vi "To Generic.vi"(8 "error in (no error)":errorcluster, 11 "NI DMM Calibration Data in":refnum<class "NI DMM Calibration Data.lvclass">) -> (0 "error out":errorcluster, 2 "Generic Data":refnum<class "Generic Data.lvclass">[](array[class]), 3 "Data Name":string[](array[string]))   [LabVIEW 2020, in "NI DMM Driver.lvlib" / "NI DMM Calibration Data.lvclass"]
doc: "Present private data as an array of named generic data elements."
uses:
  NI DMM Calibration Data.lvclass
  PPL/HDH.Data.Generic.lvlibp/Generic Data/Generic Data.lvclass
  NI DMM Calibration Data.lvclass/NI DMM Calibration Data.ctl
  PPL/HDH.Data.Generic.lvlibp/Generic Data/Time Stamp/Time Stamp.lvclass
  C:/Current projects/WS/PPL/HDH.Data.Generic.lvlibp/Generic Data/Generic Data.lvclass
  PPL/HDH.Data.Generic.lvlibp/Generic Data/String/String.lvclass
  PPL/HDH.Data.Generic.lvlibp/Generic Data/Boolean/Boolean.lvclass
  PPL/HDH.Data.Generic.lvlibp/Generic Data/Double/Double.lvclass
  PPL/HDH.Data.Generic.lvlibp/Data.lvclass
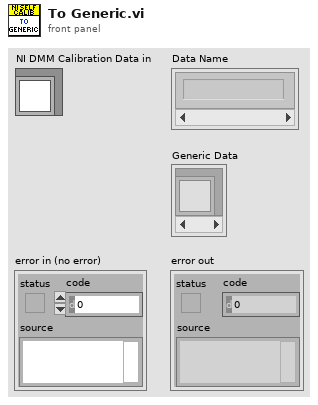
[diagram p1: front panel]
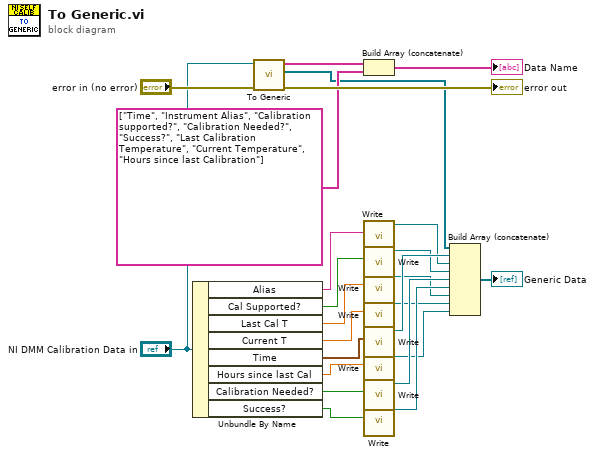
[diagram p0: block diagram]
diagram:
  n1 = Unbundle By Name("NI DMM Calibration Data in") -> ("Alias"=w13:string, "Cal Supported?"=w14:bool, "Last Cal T"=w6:dbl, "Current T"=w4:dbl, "Time"=w16:timestamp, "Hours since last Cal"=w2:dbl, "Calibration Needed?"=w10:bool, "Success?"=w9:bool)
  n2 = call-parent "To Generic.vi"("error in (no error)"="error in (no error)", "Data in"="NI DMM Calibration Data in") -> ("error out"=→"error out":errorcluster, "Generic Data"=w19:refnum<class "Generic Data.lvclass">[], "Data Name"=w23:string[])  [unwired: 7 in]
  n3 = Build Array (concatenate)(w23, string[] ["Time", "Instrument Alias", "Calibration supported?", "Calibration Needed?", "Success?", "Last Calibration Temperature", "Current Temperature", "Hours since last Calibration"] ("array")) -> (→"Data Name":string[])
  n4 = call "Write.vi"("String"=w13) -> ("String out"=w12:refnum<class "String.lvclass">)  [unwired: 10 in]
  n5 = call "Write.vi"("Boolean"=w14) -> ("Boolean out"=w11:refnum<class "Boolean.lvclass">)  [unwired: 10 in]
  n6 = call "Write.vi"("Double"=w6) -> ("Double out"=w5:refnum<class "Double.lvclass">)  [unwired: 10 in]
  n7 = call "Write.vi"("Double"=w4) -> ("Double out"=w3:refnum<class "Double.lvclass">)  [unwired: 10 in]
  n8 = call "Write.vi"("Time Stamp"=w16) -> ("Time Stamp out"=w15:refnum<class "Time Stamp.lvclass">)  [unwired: 10 in]
  n9 = call "Write.vi"("Double"=w2) -> ("Double out"=w1:refnum<class "Double.lvclass">)  [unwired: 10 in]
  n10 = call "Write.vi"("Boolean"=w10) -> ("Boolean out"=w8:refnum<class "Boolean.lvclass">)  [unwired: 10 in]
  n11 = call "Write.vi"("Boolean"=w9) -> ("Boolean out"=w7:refnum<class "Boolean.lvclass">)  [unwired: 10 in]
  n12 = Build Array (concatenate)(w19, w15, w12, w11, w8, w7, w5, w3, w1) -> (→"Generic Data":refnum<class "Generic Data.lvclass">[])
